vi "Send DB Data.vi"(0 "error in":errorcluster) -> ()   [LabVIEW 2012]
uses:
  Systems/Cannon/Cannon Global Data.vi
  Systems/Conveyer Belt/Conveyer Belt Global Data.vi
  Systems/Drive/Or David (Drive Global Data).vi
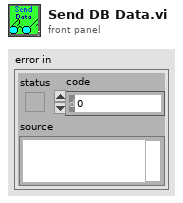
[diagram p1: front panel]
types:
  T1 = cluster{"Horizontal Belt":dbl, "Vertical Belt":dbl, "MS":bool}
  T2 = cluster{"Throttle":dbl, "RPM":dbl, "Motor VBus":dbl}
  T3 = typedef "WPI_SolenoidValue.ctl" = enum16{"Off", "On", "Forward", "Reverse"}
  T4 = cluster{"Shifter?":bool, "Axisses":dbl[], "Shifter Value":T3}
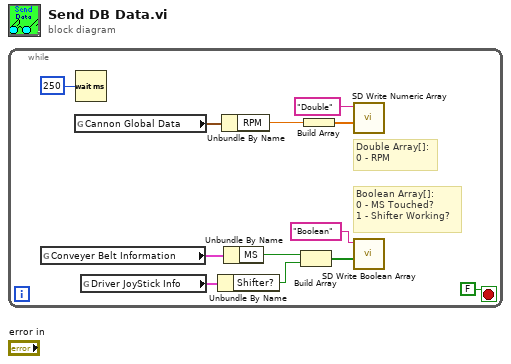
[diagram p0: block diagram]
diagram:
  n1 = while {
    stop <- FALSE stop-if-true
    # "Boolean Array[]:\n0 - MS Touched?\n1 - Shifter Working?"
    # "Double Array[]:\n0 - RPM"
    n2 = global read "Conveyer Belt Global Data.vi" "Conveyer Belt Information"() -> (w7:T1)
    n3 = global read "Cannon Global Data.vi" "Cannon Global Data"() -> (w10:T2)
    n4 = Wait (ms)(milliseconds to wait=u32 250) -> ()  [unwired: 1 out]
    n5 = global read "Or David (Drive Global Data).vi" "Driver JoyStick Info"() -> (w6:T4)
    n6 = Unbundle By Name(w6) -> ("Shifter?"=w4:bool)
    n7 = Unbundle By Name(w10) -> ("RPM"=w9:dbl)
    n8 = Unbundle By Name(w7) -> ("MS"=w5:bool)
    n9 = Build Array(w5, w4) -> (w3:bool[])
    n10 = Build Array(w9) -> (w8:dbl[])
    n11 = call <vilib>:"SD Write Numeric Array.vi"("Numeric Array"=w8, "Name"="Double") -> ()  [unwired: 8 in, 2 out]
    n12 = call <vilib>:"SD Write Boolean Array.vi"("Boolean Array"=w3, "Name"="Boolean") -> ()  [unwired: 8 in, 2 out]
  }
